vi "Average Pre Trigger Data.vi"(10 "Pretrigger points":dbl, 11 "Averaged data in":waveform(dbl)) -> (3 "Averaged data out":waveform(dbl))   [LabVIEW 2017, in "Scope.lvlib"]
uses:
  Scope.lvlib
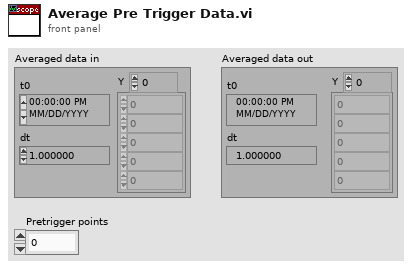
[diagram p1: front panel]
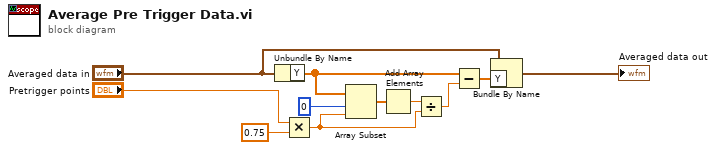
[diagram p0: block diagram]
diagram:
  n1 = Unbundle By Name("Averaged data in") -> ("Y"=w8:dbl[])
  n2 = Multiply(x="Pretrigger points", y=0.75) -> (x*y=w1:dbl)
  n3 = Array Subset(array=w8, index=0, length=w1) -> (w2:dbl[])
  n4 = Add Array Elements(numeric array=w2) -> (sum=w3:dbl)
  n5 = Divide(x=w3, y=w1) -> (x/y=w4:dbl)
  n6 = Subtract(x=w8, y=w4) -> (x-y=w9:dbl[])
  n7 = Bundle By Name(cluster="Averaged data in", "Y"=w9) -> (→"Averaged data out":waveform(dbl))
